vi "Pattern Matching.vi"() -> ()   [LabVIEW 2014]
doc: "This example shows how to use the color pattern matching tools in NI Vision.\n\nYou use color pattern matching to locate known reference or fiducial patterns in an image quickly. Pattern matching is the key to many applications. Color pattern matching can provide your application with information about the presence or absence, number, and location of the model within an image.\n\nYou use color pattern matching in the following three general applications areas:\n\n* Alignment -- Determine the position and orientation of a known object by locating features. You use the features as points of reference on the object.\n\n* Gauging -- Measure lengths, diameters, angles, and other critical dimensions. If the measurements fall outside of set tolerance levels, the component is rejected. You sometimes use gauging in-line with the manufacturing process and off-line. If you make the measurements off-line, a sample of components is used to determine the quality of a lot or batch of manufactured components.\n\n* Inspection -- Detect simple flaws, such as missing parts or unreadable printing."
uses:
  <vilib>/vision/NI_Vision_Development_Module.lvlib
panel:
  out "Number of Matches":i32
  out "Results":T1(array[cluster]) {"Score" format="%.1f"; "Position"."Y" format="%.2g"; "Position"."X" format="%.2g"}
  in  "Max # of Matches":i32=5
  in  "Minimum Score":sgl=700.0
  out "Template":T2(plugin-control)
  in  "Stop":bool
  out "Image":T2(plugin-control)
  # "Overview: Demonstrates how to perform Color Pattern Matching using two steps that include learning the color pattern template defined by a Region of Interest (ROI) and then matching the learned template in the image.\nRequirements: Vision Development Software.\nInstructions:\n1. Run the VI.\n2. Draw a ROI in the image to define the template. The learned template is displayed in the Template display and the match results are overlaid on the Image display."
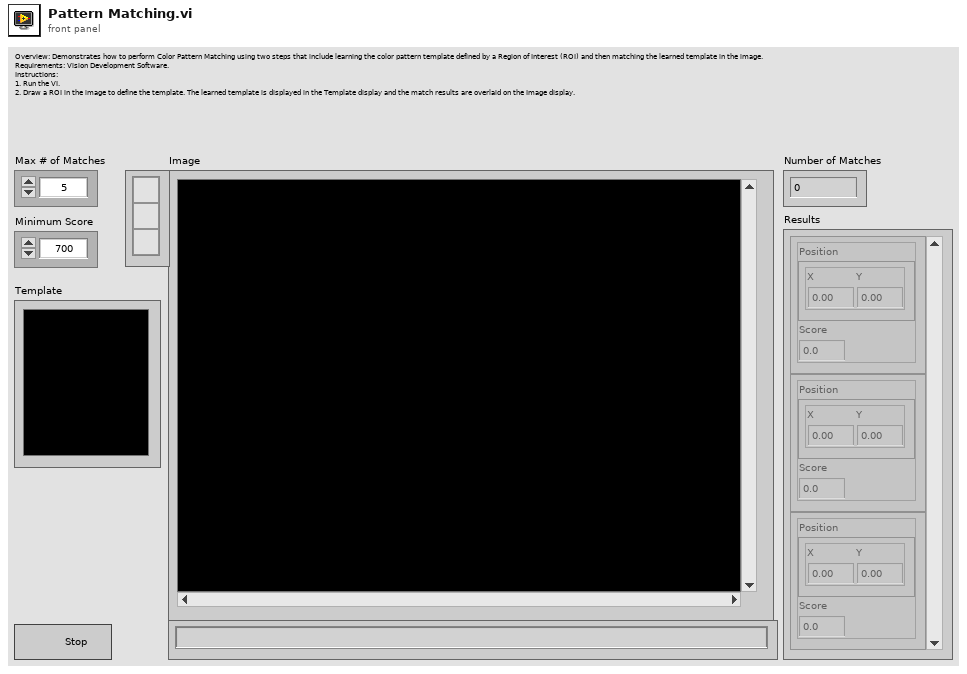
[diagram p1: front panel]
types:
  T1 = cluster{"Position":cluster{"X":dbl, "Y":dbl}, "Score":sgl}[]
  T2 = typedef "IMAQ Image.ctl" = refnum<image>
  T3 = typedef "Image Type" = u32
  T4 = typedef "IMAQ Rectangle" = cluster{"Left":i32, "Top":i32, "Right":i32, "Bottom":i32, "Rotation":dbl}
  T5 = typedef "ROI Descriptor" = cluster{"Global Rectangle":i32[], "Contours":cluster{"ID":enum32{"External", "Internal"}, "Type":u32, "Coordinates":i32[]}[]}
  T6 = cluster{"Max # of Matches":i32, "Minimum Score":sgl}
  T7 = cluster{"Position":cluster{"x":sgl, "y":sgl}, "Angle":sgl, "Scale":sgl, "Score":sgl, "Bounding Box":cluster{"x":sgl, "y":sgl}[]}[]
  T8 = cluster{"Position":cluster{"x":sgl, "y":sgl}, "Score":sgl}
  T9 = cluster{i32[], cluster{"Contour Type":u32, "ROI Type":u32, i32[]}[]}
  T10 = cluster{"Global Rectangle":i32[], "Contours":cluster{"Contour Type":u32, "ROI Type":u32, "Points":i32[]}[]}
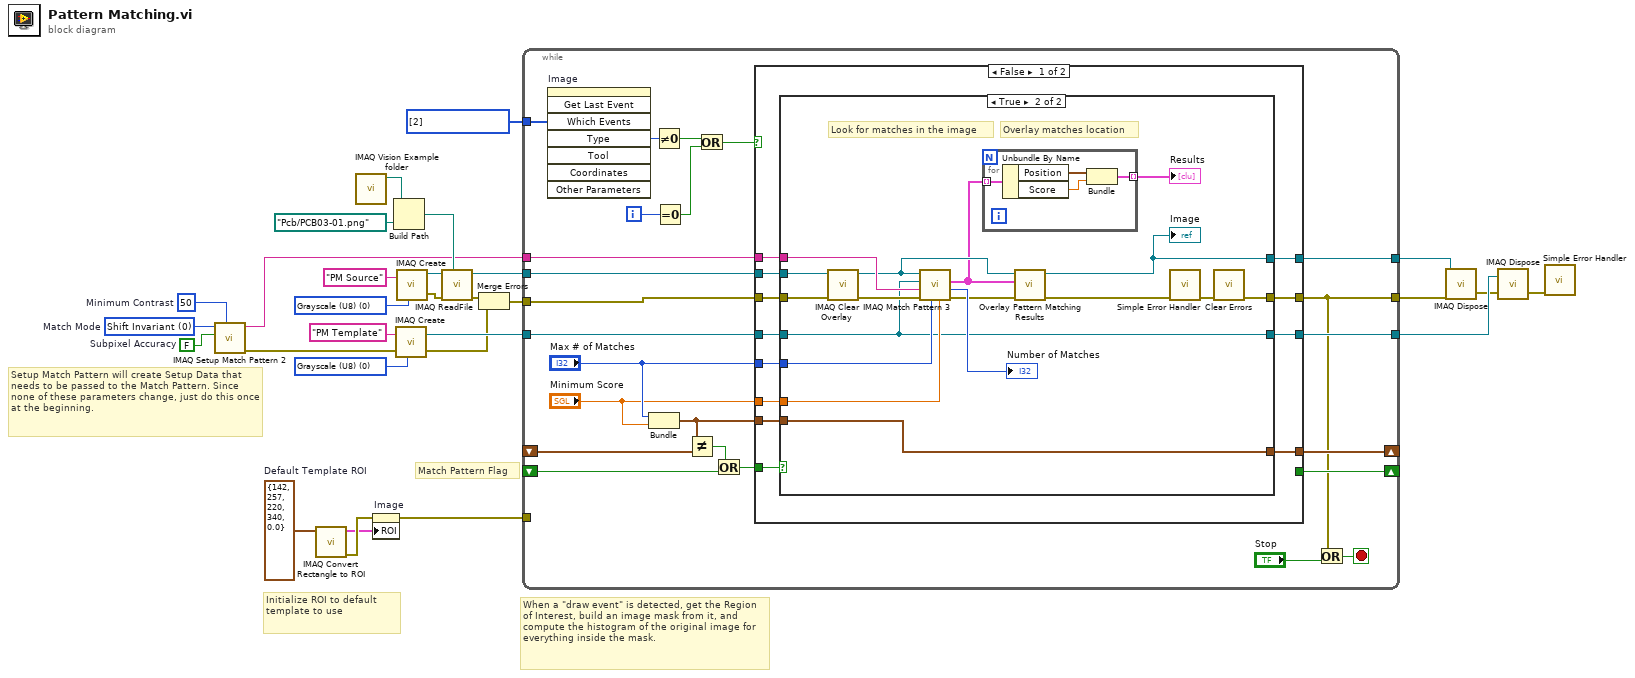
[diagram p0: block diagram]
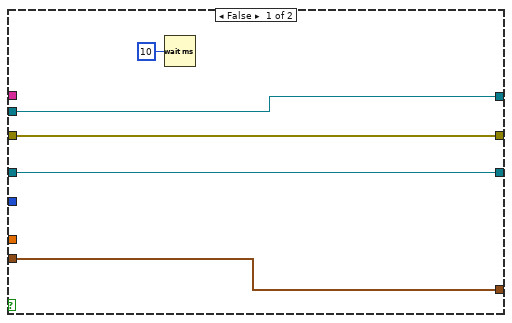
[diagram p2: hidden frame]
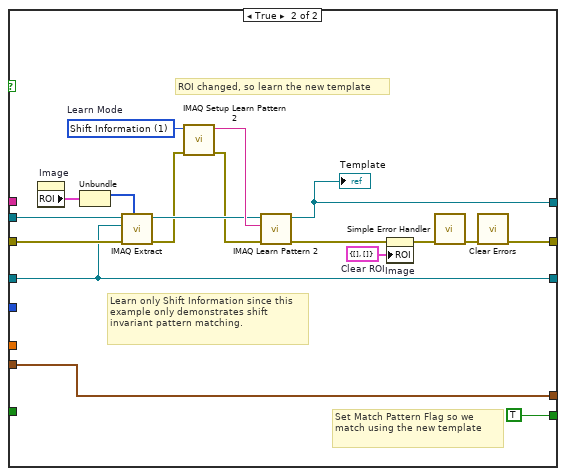
[diagram p3: hidden frame]
diagram:
  w1 = FALSE  # Subpixel Accuracy
  w2 = u16 0 items=["Shift Invariant", "Rotation Invariant"]  # Match Mode
  w5 = 50  # Minimum Contrast
  w17 = T3 0 items=["Grayscale (U8)", "Grayscale (I16)", "Grayscale (SGL)", "Complex (CSG)", "RGB (U32)", "HSL (U32)", "RGB (U64)", "Grayscale (U16)"] ("Image Type")
  w18 = T3 0 items=["Grayscale (U8)", "Grayscale (I16)", "Grayscale (SGL)", "Complex (CSG)", "RGB (U32)", "HSL (U32)", "RGB (U64)", "Grayscale (U16)"] ("Image Type")
  w23 = i32[] [2] items=["No Event"=0, "Click Event"=1, "Draw Event"=2, "Size Event"=4, "Scroll Event"=5, "Double Click Event"=8] ("Which Events")
  w25 = T4 {"Left"=142, "Top"=257, "Right"=220, "Bottom"=340, "Rotation"=0.0}  # Default Template ROI
  # "Setup Match Pattern will create Setup Data that needs to be passed to the Match Pattern. Since none of these parameters change, just do this once at the beginning."
  # "Initialize ROI to default template to use"
  # "When a \"draw event\" is detected, get the Region of Interest, build an image mask from it, and compute the histogram of the original image for everything inside the mask."
  # "Match Pattern Flag"
  n1 = call "IMAQ Setup Match Pattern 2"("Minimum Contrast"=w5, "Subpixel Accuracy"=w1, "Match Mode"=w2) -> ("error out"=w4:errorcluster, "Match Pattern Setup Data"=w3:string)  [unwired: 7 in]
  n2 = call "IMAQ Convert Rectangle to ROI"("Rectangle"=w25) -> ("error out"=w13:errorcluster, "ROI Descriptor"=w7:T5)  [unwired: 8 in]
  n3 = call "IMAQ Vision Example folder.vi"() -> ("Example Image Path"=w28:path)  [unwired: 11 in]
  n4 = property on="Image" class="ImageControl"(error in=w13, "ROI"=w7) -> (error out=w6:errorcluster)  [unwired: 1 in, 1 out]
  n5 = Build Path(base path=w28, name or relative path=path "Pcb/PCB03-01.png") -> (appended path=w24:path)
  n6 = call "IMAQ Create"("Image Name"="PM Template", "Image Type"=w17, "error in (no error)"=w4) -> ("New Image"=w22:T2, "error out"=w11:errorcluster)  [unwired: 2 in]
  n7 = call "IMAQ Create"("Image Name"="PM Source", "Image Type"=w18) -> ("New Image"=w9:T2, "error out"=w14:errorcluster)  [unwired: 3 in]
  n8 = call "IMAQ ReadFile"("File Path"=w24, "error in (no error)"=w14, "Image"=w9) -> ("error out"=w12:errorcluster, "Image Out"=w8:T2)  [unwired: 4 in, 3 out]
  n9 = Merge Errors(w12, w11) -> (w10:errorcluster)
  n10 = while {
    tunnel: w8 -> [w43]
    tunnel: w23 -> [w53]
    tunnel: w22 -> [w42]
    tunnel: w10 -> [w47]
    shift-right: [w41] -> _
    shift-left: _ -> [w34]
    shift-right: [w46] -> _
    shift-left: _ -> [w45]
    tunnel: [w39] -> w21
    tunnel: [w40] -> w20
    tunnel: [w32] -> w19
    tunnel: w6 -> [_]
    tunnel: w3 -> [w36]
    i -> [w50]
    stop <- w30 stop-if-true
    n11 = invoke on="Image" class="ImageControl" method="Get Last Event"("Which Events"=w53) -> ("Type"=w52:i32)  [unwired: 7 in, 7 out]
    n12 = Bundle("Max # of Matches"="Max # of Matches", "Minimum Score"="Minimum Score") -> (w35:T6)  [unwired: 1 in]
    n13 = Not Equal To 0?(x=w52) -> (x != 0?=w51:bool)
    n14 = Equal To 0?(x=w50) -> (x = 0?=w49:bool)
    n15 = Not Equal?(x=w35, y=w34) -> (x != y?=w33:bool)
    n16 = Or(x=w51, y=w49) -> (x .or. y?=w48:bool)
    n17 = Or(x=w33, y=w45) -> (x .or. y?=w44:bool)
    n18 = case shown="False" w48 {
      tunnel: w43 -> [w63 w101]
      tunnel: w47 -> [w62 w100]
      tunnel: w42 -> [w61 w94]
      tunnel: [_ TRUE] -> w46
      tunnel: w44 -> [w65 _]
      tunnel: w35 -> [w64 w93]
      tunnel: [w60 w97] -> w32
      tunnel: [w59 w93] -> w41
      tunnel: [w58 w94] -> w40
      tunnel: [w57 w95] -> w39
      tunnel: "Max # of Matches" -> [w56 _]
      tunnel: "Minimum Score" -> [w55 _]
      tunnel: w36 -> [w54 _]
      frame False {
        n19 = case shown="True" w65 {
          tunnel: w64 -> [w68 w85]
          tunnel: w63 -> [w66 w87]
          tunnel: w62 -> [w70 w86]
          tunnel: w61 -> [w67 w76]
          tunnel: [w70 w83] -> w60
          tunnel: [w68 w85] -> w59
          tunnel: [w67 w76] -> w58
          tunnel: [w66 w75] -> w57
          tunnel: w56 -> [_ w81]
          tunnel: w55 -> [_ w80]
          tunnel: w54 -> [_ w79]
          frame False {
            n20 = Wait (ms)(milliseconds to wait=u32 10) -> ()  [unwired: 1 out]
          }
          frame True {
            # "Overlay matches location"
            # "Look for matches in the image"
            n21 = call "IMAQ Clear Overlay"("error in (no error)"=w86, "Image"=w87) -> ("error out"=w82:errorcluster, "Image Out"=w73:T2)  [unwired: 8 in]
            n22 = call "IMAQ Match Pattern 3"("Minimum Match Score"=w80, "Number of Matches Requested"=w81, "error in (no error)"=w82, "Match Pattern Setup Data"=w79, "Template Image"=w76, "Image"=w73) -> ("error out"=w71:errorcluster, "Number of Matches"=→"Number of Matches":i32, "Matches"=w72:T7)  [unwired: 3 in]
            n23 = for {
              tunnel: w72 -> [w91] mode=indexing
              tunnel: [w88] -> w78 mode=indexing
              n24 = Unbundle By Name(w91) -> ("Position"=w90:cluster{"x":sgl, "y":sgl}, "Score"=w89:sgl)
              n25 = Bundle("Position"=w90, "Score"=w89) -> (w88:T8)  [unwired: 1 in]
            }
            "Results" <- w78
            n26 = call "Overlay Pattern Matching Results.vi"("error in"=w71, "Matches"=w72, "Image"=w73) -> ("error out"=w74:errorcluster, "Image Out"=w75:T2)  [unwired: 7 in]
            "Image" <- w75
            n27 = call <vilib>:"Simple Error Handler.vi"("error in (no error)"=w74) -> ("error out"=w84:errorcluster)  [unwired: 4 in, 4 out]
            n28 = call <vilib>:"Clear Errors.vi"("error in (no error)"=w84) -> ("error out"=w83:errorcluster)  [unwired: 5 in, 1 out]
          }
        }
      }
      frame True {
        w92 = u16 1 items=["All", "Shift Information", "Rotation Information"]  # Learn Mode
        w102 = T9 {[], []}  # Clear ROI
        # "Set Match Pattern Flag so we match using the new template"
        # "Learn only Shift Information since this example only demonstrates shift invariant pattern matching."
        # "ROI changed, so learn the new template"
        n29 = property on="Image" class="ImageControl"() -> ("ROI"=w104:T10)  [unwired: 2 in, 2 out]
        n30 = Unbundle(w104) -> ("Global Rectangle"=w109:i32[])  [unwired: 1 out]
        n31 = call "IMAQ Extract"("Optional Rectangle"=w109, "error in (no error)"=w100, "Image Dst"=w94, "Image Src"=w101) -> ("error out"=w106:errorcluster, "Image Dst Out"=w107:T2)  [unwired: 6 in]
        n32 = call "IMAQ Setup Learn Pattern 2"("error in (no error)"=w106, "Learn Mode"=w92) -> ("error out"=w105:errorcluster, "Learn Pattern Setup Data"=w108:string)  [unwired: 8 in]
        n33 = call "IMAQ Learn Pattern 2"("error in (no error)"=w105, "Learn Pattern Setup Data"=w108, "Image"=w107) -> ("error out"=w96:errorcluster, "Template Image Out"=w95:T2)  [unwired: 7 in]
        "Template" <- w95
        n34 = property on="Image" class="ImageControl"(error in=w96, "ROI"=w102) -> (error out=w103:errorcluster)  [unwired: 1 in, 1 out]
        n35 = call <vilib>:"Simple Error Handler.vi"("error in (no error)"=w103) -> ("error out"=w98:errorcluster)  [unwired: 4 in, 4 out]
        n36 = call <vilib>:"Clear Errors.vi"("error in (no error)"=w98) -> ("error out"=w97:errorcluster)  [unwired: 5 in, 1 out]
      }
    }
    n37 = Or(x=w32, y="Stop") -> (x .or. y?=w30:bool)
  }
  n38 = call "IMAQ Dispose"("Image"=w21, "error in (no error)"=w19) -> ("error out"=w16:errorcluster)  [unwired: 4 in]
  n39 = call "IMAQ Dispose"("Image"=w20, "error in (no error)"=w16) -> ("error out"=w15:errorcluster)  [unwired: 4 in]
  n40 = call <vilib>:"Simple Error Handler.vi"("error in (no error)"=w15) -> ()  [unwired: 4 in, 5 out]
